vi "InitPrefMetadataFromPrefCluster.vi"(8 "error in (no error)":errorcluster, 11 "Preferences in":refnum<class "SetListPrefs.lvclass">) -> (0 "error out":errorcluster, 3 "Preferences out":refnum<class "SetListPrefs.lvclass">)   [LabVIEW 2013, in "SetListPrefs.lvclass"]
doc: "Initializes list of Preference Names and Preference Descriptions from the cluster"
uses:
  SetListPrefs.lvclass
  PrefCluster.ctl
  <vilib>/Utility/miscctls.llb/LVRectTypeDef.ctl
  SetListPrefs.lvclass/SetListPrefs.ctl
panel:
  out "PrefCluster":T1
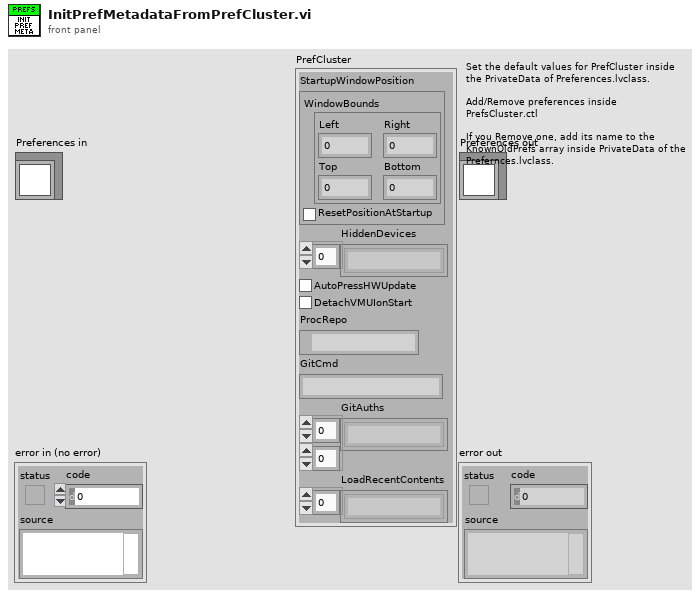
[diagram p1: front panel]
types:
  T1 = typedef "SetListPrefs.lvclass/PrefCluster.ctl" = cluster{"StartupWindowPosition":cluster{"WindowBounds":T2, "ResetPositionAtStartup":bool}, "HiddenDevices":string[], "AutoPressHWUpdate":bool, "DetachVMUIonStart":bool, "ProcRepo":path, "GitCmd":string, "GitAuths":string[][], "LoadRecentContents":string[]}
  T2 = typedef "LVRectTypeDef.ctl" = cluster{"Left":i16, "Top":i16, "Right":i16, "Bottom":i16}
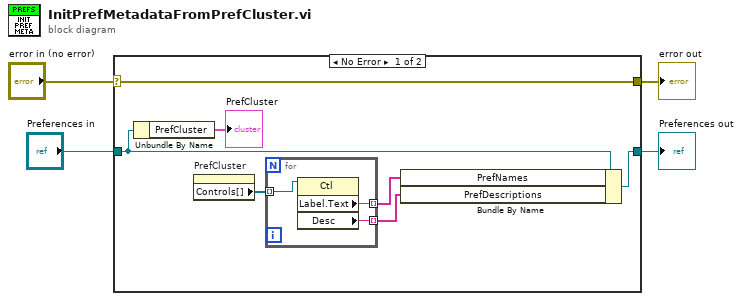
[diagram p0: block diagram]
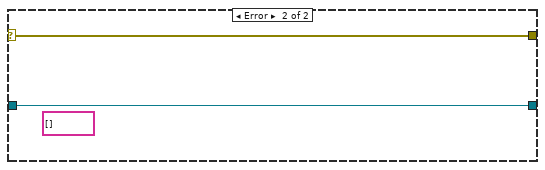
[diagram p2: hidden frame]
diagram:
  n1 = case shown="No Error" "error in (no error)" {
    selector: "error in (no error)" -> [w11 w16]
    tunnel: [w11 w16] -> w3
    tunnel: [w7 w15] -> w1
    tunnel: "Preferences in" -> [w8 w15]
    frame No Error {
      n2 = Unbundle By Name(w8) -> ("PrefCluster"=→"PrefCluster":T1)
      n3 = property on="PrefCluster" class="Clust (strict)"() -> ("Controls[]"=w9:refnum<vi>[])  [unwired: 2 in, 2 out]
      n4 = for {
        tunnel: w9 -> [w14] mode=indexing
        tunnel: [w13] -> w6 mode=indexing
        tunnel: [w12] -> w5 mode=indexing
        n5 = property class="Ctl"(reference=w14) -> ("Label.Text"=w13:string, "Desc"=w12:string)  [unwired: 1 in, 2 out]
      }
      n6 = Bundle By Name(cluster=w8, "PrefNames"=w6, "PrefDescriptions"=w5) -> (w7:refnum<class "SetListPrefs.lvclass">)
    }
    frame Error {
      (unwired) string[] []
    }
  }
  "error out" <- w3
  "Preferences out" <- w1
